vi "Search for Channel FIFO Index.vi"(8 "error in (no error)":errorcluster, 10 "Item Ref":T1 format="%.0x", 11 "Specified Channel Ref List":T1[](array[typedef]) format="%.0x") -> (0 "error out":errorcluster, 3 "index of element":i32)   [LabVIEW 2019, in "Ballard Arinc-429 System Explorer.lvlib"]
uses:
  Ballard Arinc-429 System Explorer.lvlib
  <vilib>/NI VeriStand/Custom Device API/Custom Device Item Ref.ctl
  <vilib>/NI VeriStand/Custom Device API/Custom Device API.lvlib
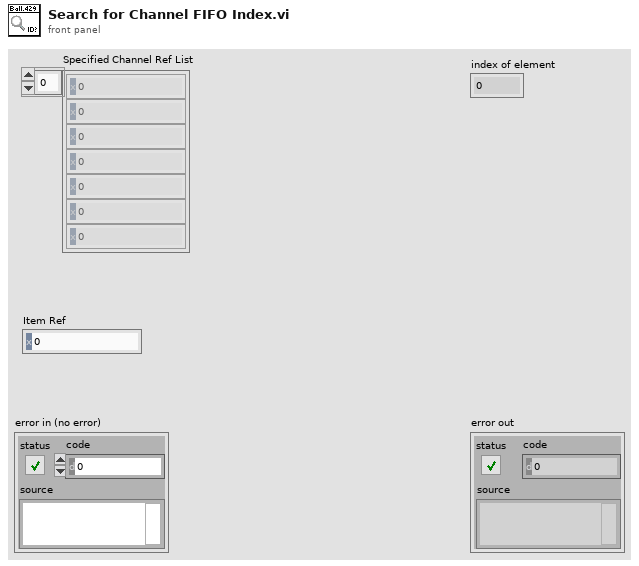
[diagram p1: front panel]
types:
  T1 = typedef "Custom Device API.lvlib/Custom Device Item Ref.ctl" = u64
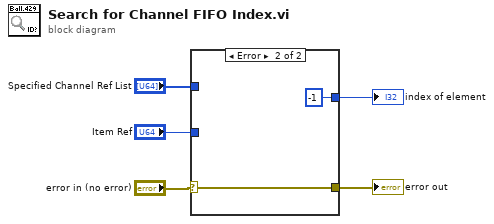
[diagram p0: block diagram]
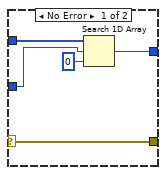
[diagram p2: hidden frame]
diagram:
  n1 = case shown="Error" "error in (no error)" {
    selector: "error in (no error)" -> [w8 w12]
    tunnel: [w8 w12] -> w4
    tunnel: [w10 -1 ("index of element")] -> w3
    tunnel: "Specified Channel Ref List" -> [w9 _]
    tunnel: "Item Ref" -> [w7 _]
    frame No Error {
      n2 = Search 1D Array(1D array=w9, element=w7, start index (0)=0) -> (index of element=w10:i32)
    }
    frame Error {
    }
  }
  "error out" <- w4
  "index of element" <- w3
